vi "Set Sart Cameras.vi"(6 "Main Camera 4":T1="dummy", 8 "error in (no error)":errorcluster, 9 "Camera 3":T1="dummy", 10 "Camera 2":T1="dummy", 11 "HIJ 4 Aligment Cams Launcher in":refnum<class "HIJ 4 Aligment Cams Launcher.lvclass">) -> (0 "error out":errorcluster, 3 "HIJ 4 Aligment Cams Launcher out":refnum<class "HIJ 4 Aligment Cams Launcher.lvclass">)   [LabVIEW 2014, in "HIJ 4 Alignment Cams App.lvlib" / "HIJ 4 Aligment Cams Launcher.lvclass"]
uses:
  HIJ 4 Aligment Cams Launcher.lvclass
  <vilib>/userdefined/High Color/IMAQdx.ctl
  HIJ 4 Alignment Cams App/HIJ 4 Alignment Cams App.lvclass
  HIJ Vision Launcher/HIJ Vision Launcher/HIJ Vision Launcher.lvclass/HIJ Vision Launcher.ctl
  HIJ 4 Alignment Cams App/HIJ 4 Alignment Cams App.lvclass/HIJ 4 Alignment Cams App.ctl
  HIJ Vision Launcher/HIJ Vision Launcher/Read HIJ Vision Camera App.vi
  HIJ 4 Alignment Cams App/Write Start Camera 2.vi
  HIJ 4 Alignment Cams App/Write Start Camera 3.vi
  HIJ 4 Alignment Cams App/Write Start Camera 4.vi
  HIJ Vision Launcher/HIJ Vision Launcher/Write HIJ Vision Camera App.vi
  Shared Code/Viewable Actor/ViewableActor/ViewableActor.lvclass
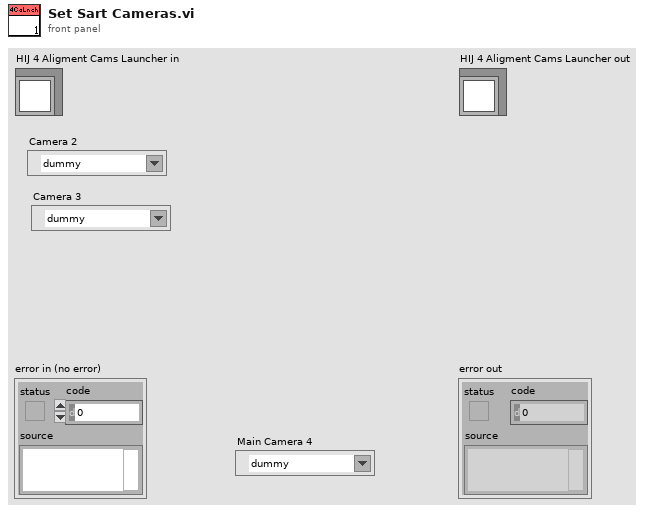
[diagram p1: front panel]
types:
  T1 = typedef "IMAQdx.ctl" = refnum<k21>
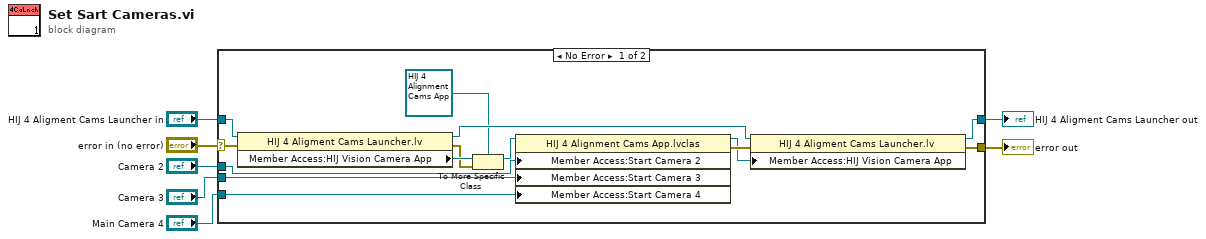
[diagram p0: block diagram]
diagram:
  n1 = case shown="No Error" "error in (no error)" {
    selector: "error in (no error)" -> [w10 w23]
    tunnel: [w9 w23] -> w6
    tunnel: [w19 w22] -> w4
    tunnel: "HIJ 4 Aligment Cams Launcher in" -> [w21 w22]
    tunnel: "Camera 2" -> [w14 _]
    tunnel: "Camera 3" -> [w13 _]
    tunnel: "Main Camera 4" -> [w12 _]
    frame No Error {
      n2 = property class="HIJ 4 Aligment Cams Launcher.lv"(reference=w21, error in=w10) -> (reference out=w20:refnum<class "HIJ 4 Aligment Cams Launcher.lvclass">, error out=w15:errorcluster, "Member Access:HIJ Vision Camera App"=w18:refnum<class "ViewableActor.lvclass">)
      n3 = To More Specific Class(target class=refnum<class "HIJ 4 Alignment Cams App.lvclass"> refnum ("HIJ 4 Alignment Cams App.lvlib:HIJ 4 Alignment Cams App.lvclass"), reference=w18, error in=w15) -> (specific class reference=w17:refnum<class "HIJ 4 Alignment Cams App.lvclass">)  [unwired: 1 out]
      n4 = property class="HIJ 4 Alignment Cams App.lvclas"(reference=w17, "Member Access:Start Camera 2"=w14, "Member Access:Start Camera 3"=w13, "Member Access:Start Camera 4"=w12) -> (reference out=w8:refnum<class "HIJ 4 Alignment Cams App.lvclass">, error out=w11:errorcluster)  [unwired: 1 in]
      n5 = property class="HIJ 4 Aligment Cams Launcher.lv"(reference=w20, error in=w11, "Member Access:HIJ Vision Camera App"=w8) -> (reference out=w19:refnum<class "HIJ 4 Aligment Cams Launcher.lvclass">, error out=w9:errorcluster)
    }
    frame Error {
    }
  }
  "error out" <- w6
  "HIJ 4 Aligment Cams Launcher out" <- w4
